vi "Dresser DXD Read from EEPROM.vi"(0 "VISA session":refnum<visa-resource-name>, 5 "DXD Address (1)":T1=1 min=1 max=99 step=1, 7 "EEPROM Read Address (0)":i32 min=0 max=255 step=1, 11 "Error In (no error)":errorcluster) -> (4 "dup VISA session":refnum<visa-resource-name>, 6 "Returned String":string, 8 "EEPROM Value":i32, 15 "Error Out":errorcluster)   [LabVIEW 2015]
doc: "This VI will read the value from the specified EEPROM Address of the Dresser DXD Series pressure transducer.\n\nWritten by:\nBLOOMY CONTROLS, INC\nWINDSOR, CT 06095, USA\n860-298-9925\nwww.bloomy.com\nV2.0.0\nMay, 2002"
uses:
  Type Defs/DXD Address.ctl
panel:
  # "For instructions on the use of this VI, press Ctrl+H to display the help window and move the mouse over the icon, controls, and indicators"
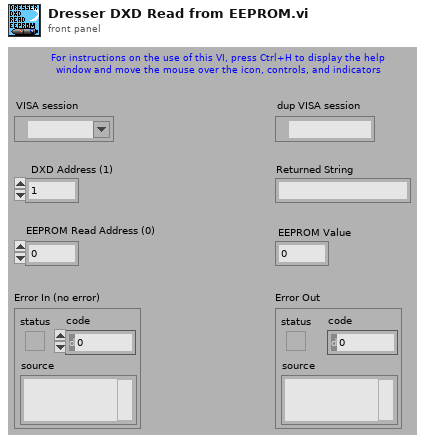
[diagram p1: front panel]
types:
  T1 = typedef "DXD Address.ctl" = i32
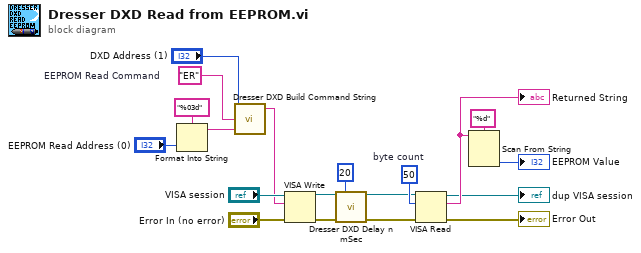
[diagram p0: block diagram]
diagram:
  w14 = u32 50  # byte count
  w16 = "ER"  # EEPROM Read Command
  n1 = Format Into String(format string="%03d" ("Format String"), "EEPROM Read Address (0)") -> (resulting string=w11:string)  [unwired: 2 in, 1 out]
  n2 = call "Dresser DXD Build Command String.vi"("Input Value (\"\")"=w11, "Command Mnemonic (\"\")"=w16, "DXD Address (1)"="DXD Address (1)") -> ("Command String"=w15:string)  [unwired: 2 in]
  n3 = VISA Write(VISA resource name="VISA session", write buffer=w15, error in (no error)="Error In (no error)") -> (VISA resource name out=w6:refnum<visa-resource-name>, error out=w5:errorcluster)  [unwired: 1 out]
  n4 = call "Dresser DXD Delay n mSec.vi"("VISA session"=w6, "Milliseconds to Wait (0)"=u32 20, "Error In (no error)"=w5) -> ("dup VISA session"=w7:refnum<visa-resource-name>, "Error Out"=w8:errorcluster)  [unwired: 11 in]
  n5 = VISA Read(VISA resource name=w7, byte count=w14, error in (no error)=w8) -> (VISA resource name out=→"dup VISA session":refnum<visa-resource-name>, read buffer=w3:string, error out=→"Error Out":errorcluster)  [unwired: 1 out]
  "Returned String" <- w3
  n6 = Scan From String(format string="%d" ("Format String"), input string=w3) -> (output 1=→"EEPROM Value":i32)  [unwired: 3 in, 3 out]
